vi "setAllChannels.vi"(8 "error in (no error)":errorcluster, 9 "allChannelProperties":variant, 11 "Instrument.Amplifier in":refnum<class "Instrument.Amplifier.lvclass">) -> (0 "error out":errorcluster, 3 "Instrument.Amplifier out":refnum<class "Instrument.Amplifier.lvclass">)   [LabVIEW 2019, in "Instrument.Amplifier.lvclass"]
uses:
  Instrument.Amplifier.lvclass
  Amplifier.Commands--Enum.ctl
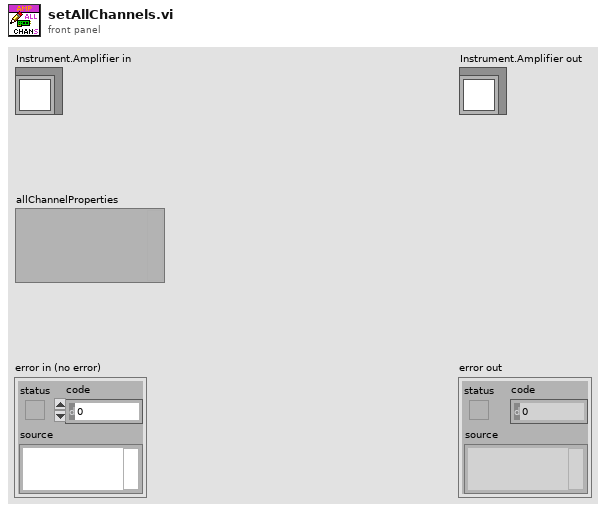
[diagram p1: front panel]
types:
  T1 = typedef "Instrument.Amplifier.lvclass/Amplifier.Commands--Enum.ctl" = enum16{"getChannel", "getAllChannels", "setChannel", "setAllChannels"}
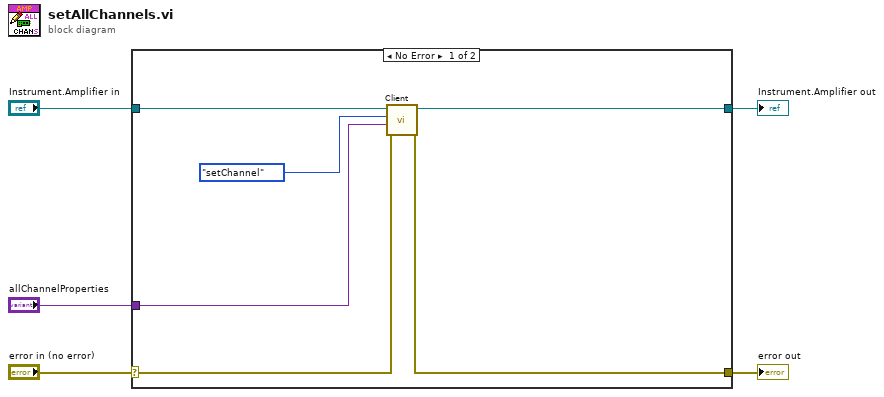
[diagram p0: block diagram]
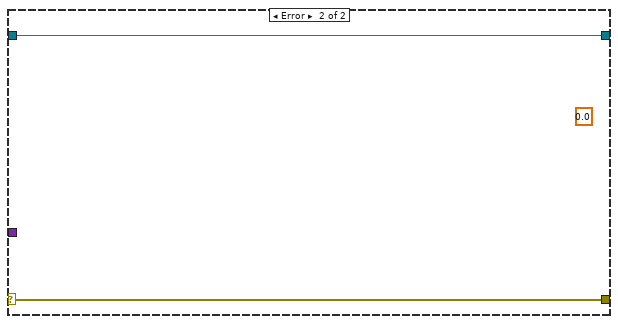
[diagram p2: hidden frame]
diagram:
  n1 = case shown="No Error" "error in (no error)" {
    selector: "error in (no error)" -> [w8 w13]
    tunnel: [w7 w13] -> w4
    tunnel: [w11 w12] -> w2
    tunnel: "Instrument.Amplifier in" -> [w9 w12]
    tunnel: "allChannelProperties" -> [w10 _]
    frame No Error {
      n2 = call-dynamic "Client.vi"("error in (no error)"=w8, "Data in"=w10, "Command in"=Amplifier.Commands--Enum."setChannel" ("Commands"), "Instrument in"=w9) -> ("error out"=w7:errorcluster, "Instrument out"=w11:refnum<class "Instrument.Amplifier.lvclass">)  [unwired: 4 in, 2 out]
    }
    frame Error {
      (unwired) 0.0 ("Data out")
    }
  }
  "error out" <- w4
  "Instrument.Amplifier out" <- w2
